vi "Generate_Report.vi"() -> ()   [LabVIEW 2019]
uses:
  <vilib>/Utility/NIReport.llb/Report Type.ctl
  <vilib>/Utility/NIReport.llb/image depth.ctl
  <vilib>/Utility/NIReport.llb/Append Report Text (str wrap).vi
  <vilib>/Utility/NIReport.llb/NI_report.lvclass
  <vilib>/Utility/NIReport.llb/NI_ReportGenerationCore.lvlib
  <vilib>/Utility/NIReport.llb/Word/NI_Word.lvclass
panel:
  in  "error in":errorcluster
  out "Sinal Tempo":cluster{"t0":dbl, "dt":dbl, "Y":dbl[]}(graph)
  out "Sinal Frequencia":dbl[](graph)
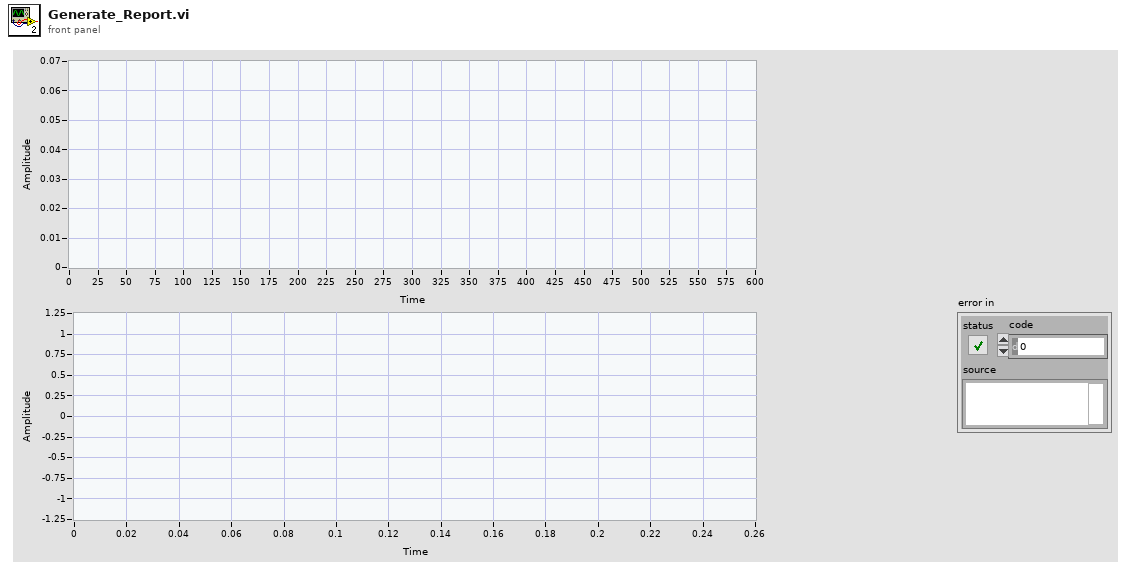
[diagram p1: front panel]
types:
  T1 = enum16{"maximized", "minimized", "normal", "no change"}
  T2 = typedef "NI_ReportGenerationCore.lvlib/Report Type.ctl" = enum16{"HTML", "Word", "Excel"}
  T3 = cluster{"position (Excel)":cluster{"row":i32, "column":i32}, "name (Excel)":string, "bookmark (Word)":string}
  T4 = typedef "NI_ReportGenerationCore.lvlib/image depth.ctl" = u16
  T5 = cluster{"position (excel)":cluster{"row":i32, "column":i32}, "name (excel)":string, "bookmark (word)":string}
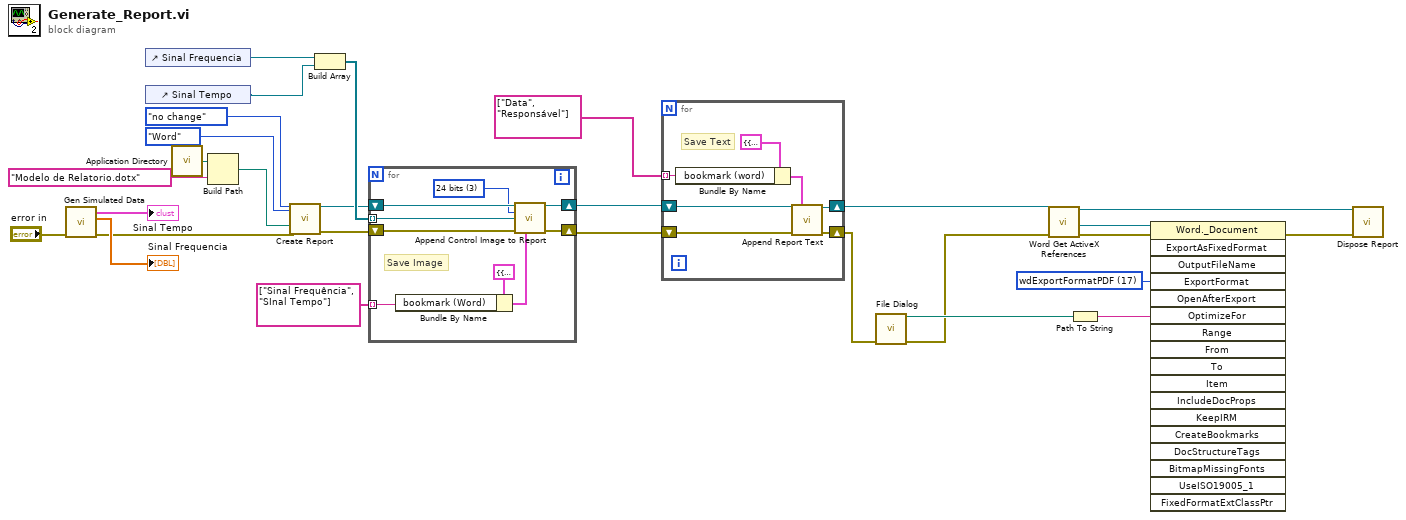
[diagram p0: block diagram]
diagram:
  w11 = 17 items=["wdExportFormatPDF"=17, "wdExportFormatXPS"=18] ("ExportFormat")
  n1 = call "Gen Simulated Data.vi"("error in (no error)"="error in") -> ("error out"=w1:errorcluster, "Sinal Frequencia"=→"Sinal Frequencia":dbl[], "Sinal Tempo"=→"Sinal Tempo":cluster{"t0":dbl, "dt":dbl, "Y":dbl[]})  [unwired: 8 in]
  n2 = control-ref of="Sinal Frequencia"() -> (w22:refnum<vi>)
  n3 = control-ref of="Sinal Tempo"() -> (w2:refnum<vi>)
  n4 = call <vilib>:"Application Directory.vi"() -> ("Application Directory"=w3:path)
  n5 = Build Path(base path=w3, name or relative path="Modelo de Relatorio.dotx") -> (appended path=w16:path)
  n6 = call <vilib>:"Create Report.vi"("window state (normal)"=T1."no change", "report type"=Report_Type."Word", "template (empty)"=w16, "error in (no error)"=w1) -> ("report out"=w18:refnum<class "NI_report.lvclass">, "error out"=w17:errorcluster)  [unwired: 10 in]
  n7 = Build Array(w22, w2) -> (w21:refnum<vi>[])
  n8 = for {
    tunnel: string[] ["Sinal Frequência", "SInal Tempo"] -> [w36] mode=indexing
    tunnel: w21 -> [w31] mode=indexing
    shift-right: [w35] -> w20
    shift-left: w18 -> [w34]
    shift-right: [w33] -> w19
    shift-left: w17 -> [w32]
    w29 = T4 3 items=["B&W", "4 bits", "8 bits", "24 bits"] ("image depth")
    # "Save Image"
    n9 = Bundle By Name(cluster=T3 {"position (Excel)"={"row"=0, "column"=0}, "name (Excel)"="", "bookmark (Word)"=""} ("MS Office parameters"), "bookmark (Word)"=w36) -> (w30:T3)
    n10 = call-dynamic "Append Control Image to Report.vi"("report in"=w34, "image depth"=w29, "ctrl reference"=w31, "error in (no error)"=w32, "MS Office parameters"=w30) -> ("report out"=w35:refnum<class "NI_report.lvclass">, "error out"=w33:errorcluster)  [unwired: 7 in, 2 out]
  }
  n11 = for {
    shift-right: [w43] -> w4
    shift-left: w20 -> [w42]
    shift-right: [w41] -> w6
    shift-left: w19 -> [w40]
    tunnel: string[] ["Data", "Responsável"] -> [w39] mode=indexing
    # "Save Text"
    n12 = Bundle By Name(cluster=T5 {"position (excel)"={"row"=0, "column"=0}, "name (excel)"="", "bookmark (word)"=""} ("MS Office parameters"), "bookmark (word)"=w39) -> (w44:T5)
    n13 = call-poly <vilib>:"Append Report Text.vi"("report in"=w42, "MS Office parameters"=w44, "error in (no error)"=w40) -> ("report out"=w43:refnum<class "NI_report.lvclass">, "error out"=w41:errorcluster)  [unwired: 9 in, 2 out]
  }
  n14 = call "File Dialog"("error in"=w6) -> ("selected path"=w7:path, "error out"=w5:errorcluster)  [unwired: 11 in, 2 out]
  n15 = call <vilib>:"Word Get ActiveX References.vi"("report in"=w4, "error in (no error)"=w5) -> ("report out"=w9:refnum<class "NI_report.lvclass">, "Word._Document"=w12:refnum<k7>, "error out"=w13:errorcluster)  [unwired: 7 in, 4 out]
  n16 = Path To String(path=w7) -> (string=w8:string)
  n17 = invoke class="Word._Document" method="ExportAsFixedFormat"(reference=w12, error in=w13, "OutputFileName"=w8, "ExportFormat"=w11) -> (error out=w10:errorcluster)  [unwired: 14 in, 17 out]
  n18 = call-dynamic "Dispose Report.vi"("report in"=w9, "error in (no error)"=w10) -> ()  [unwired: 13 in, 1 out]
